vi "Four Sensor Test.vi"() -> ()   [LabVIEW 2013]
uses:
  <vilib>/FPGAPlugInAG/sbRIO-9642/niLvFpga_Open_sbRIO-9642.vi
  <vilib>/rvi/interface/common/dynamic/niFpgaDynamicAddResources.vi
  <vilib>/rvi/interface/common/niFpgaWaitOnOcc.vi
  <vilib>/Utility/error.llb/Error Cluster From Error Code.vi
  <vilib>/rvi/errors/niLvFpgaAdjustHostInterfaceError.vi
  <vilib>/rvi/interface/nirviOpenFPGA/nirviOpenFPGA.xnode
  FPGA Bitfiles/NatesProject1_FPGATarget_FPGAConfig_gDHlPw7zMRU.lvbitx
  FPGA Config.vi
  <vilib>/rvi/interface/nirviReadWriteControl/nirviReadWriteControl.xnode
  NiFpgaLv.dll
  <vilib>/rvi/interface/Simulation/niFpgaSimulationCallBeginRW.vi
panel:
  out "Rear Sonar\nDistance\n(cm)":dbl(slide) scale=0.0..150.0
  out "Front Sonar\nDistance\n(cm)":dbl(slide) scale=0.0..150.0
  out "ModA/AI3":fxp<+/-,26,5>
  out "ModA/AI2":fxp<+/-,26,5>
  out "ModA/AI1":fxp<+/-,26,5>
  out "Front IR\nDistance\n(m)":dbl(slide) scale=0.0..1.5
  out "Rear IR\nDistance\n(m)":dbl(slide) scale=0.0..1.5
  in  "stop":bool
  out "ModA/AI0":fxp<+/-,26,5>
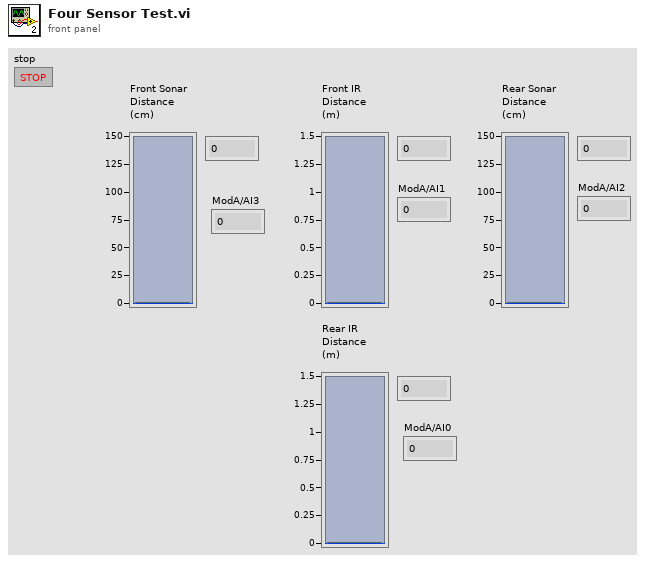
[diagram p1: front panel]
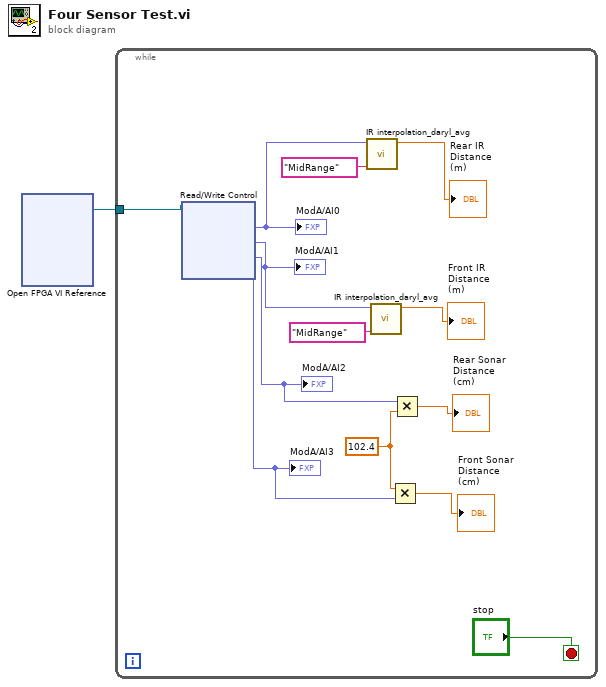
[diagram p0: block diagram]
diagram:
  n1 = xnode "Open FPGA VI Reference"() -> ("FPGA VI Reference Out"=w1:refnum<k20>)  [unwired: 2 in, 1 out]
  n2 = while {
    tunnel: w1 -> [w14]
    stop <- "stop" stop-if-true
    w6 = 102.4
    n3 = xnode "Read/Write Control"("FPGA VI Reference In"=w14) -> ("ModA/AI0"=w12:fxp<+/-,26,5>, "ModA/AI1"=w9:fxp<+/-,26,5>, "ModA/AI2"=w5:fxp<+/-,26,5>, "ModA/AI3"=w4:fxp<+/-,26,5>)  [unwired: 1 in, 2 out]
    "ModA/AI0" <- w12
    "ModA/AI1" <- w9
    "ModA/AI2" <- w5
    "ModA/AI3" <- w4
    n4 = call "IR interpolation_daryl_avg.vi"("IR Sensor Type"="MidRange", "x value"=w12) -> ("interpolation value"=→"Rear IR\nDistance\n(m)":dbl)  [unwired: 9 in]
    n5 = call "IR interpolation_daryl_avg.vi"("IR Sensor Type"="MidRange", "x value"=w9) -> ("interpolation value"=→"Front IR\nDistance\n(m)":dbl)  [unwired: 9 in]
    n6 = Multiply(x=w6, y=w4) -> (x*y=→"Front Sonar\nDistance\n(cm)":dbl)
    n7 = Multiply(x=w5, y=w6) -> (x*y=→"Rear Sonar\nDistance\n(cm)":dbl)
  }
